vi "古田户外一体站流程质控自动启动.vi"(11 "参数":T1={"是否启用仪器"=FALSE, "CODMn"={"启动测量模式"={"测量模式"=enum."水样测量"}, "确定按钮"=TRUE}, "启动模块"={"氨氮"=FALSE, "总磷"=FALSE, "总氮"=FALSE, "COD"=FALSE}, "常规启动"=FALSE, "直接启动"=FALSE}) -> ()   [LabVIEW 2016, in "质控单元.lvlib"]
uses:
  PLC/PLC.lvlib
panel:
  out "枚举 2":enum16{"初始化", "采配水启动", "等待", "配水", "排水", "结束"}(ring)
  out "枚举":enum16{"初始化", "采配水启动", "等待", "配水", "排水", "结束"}(ring)
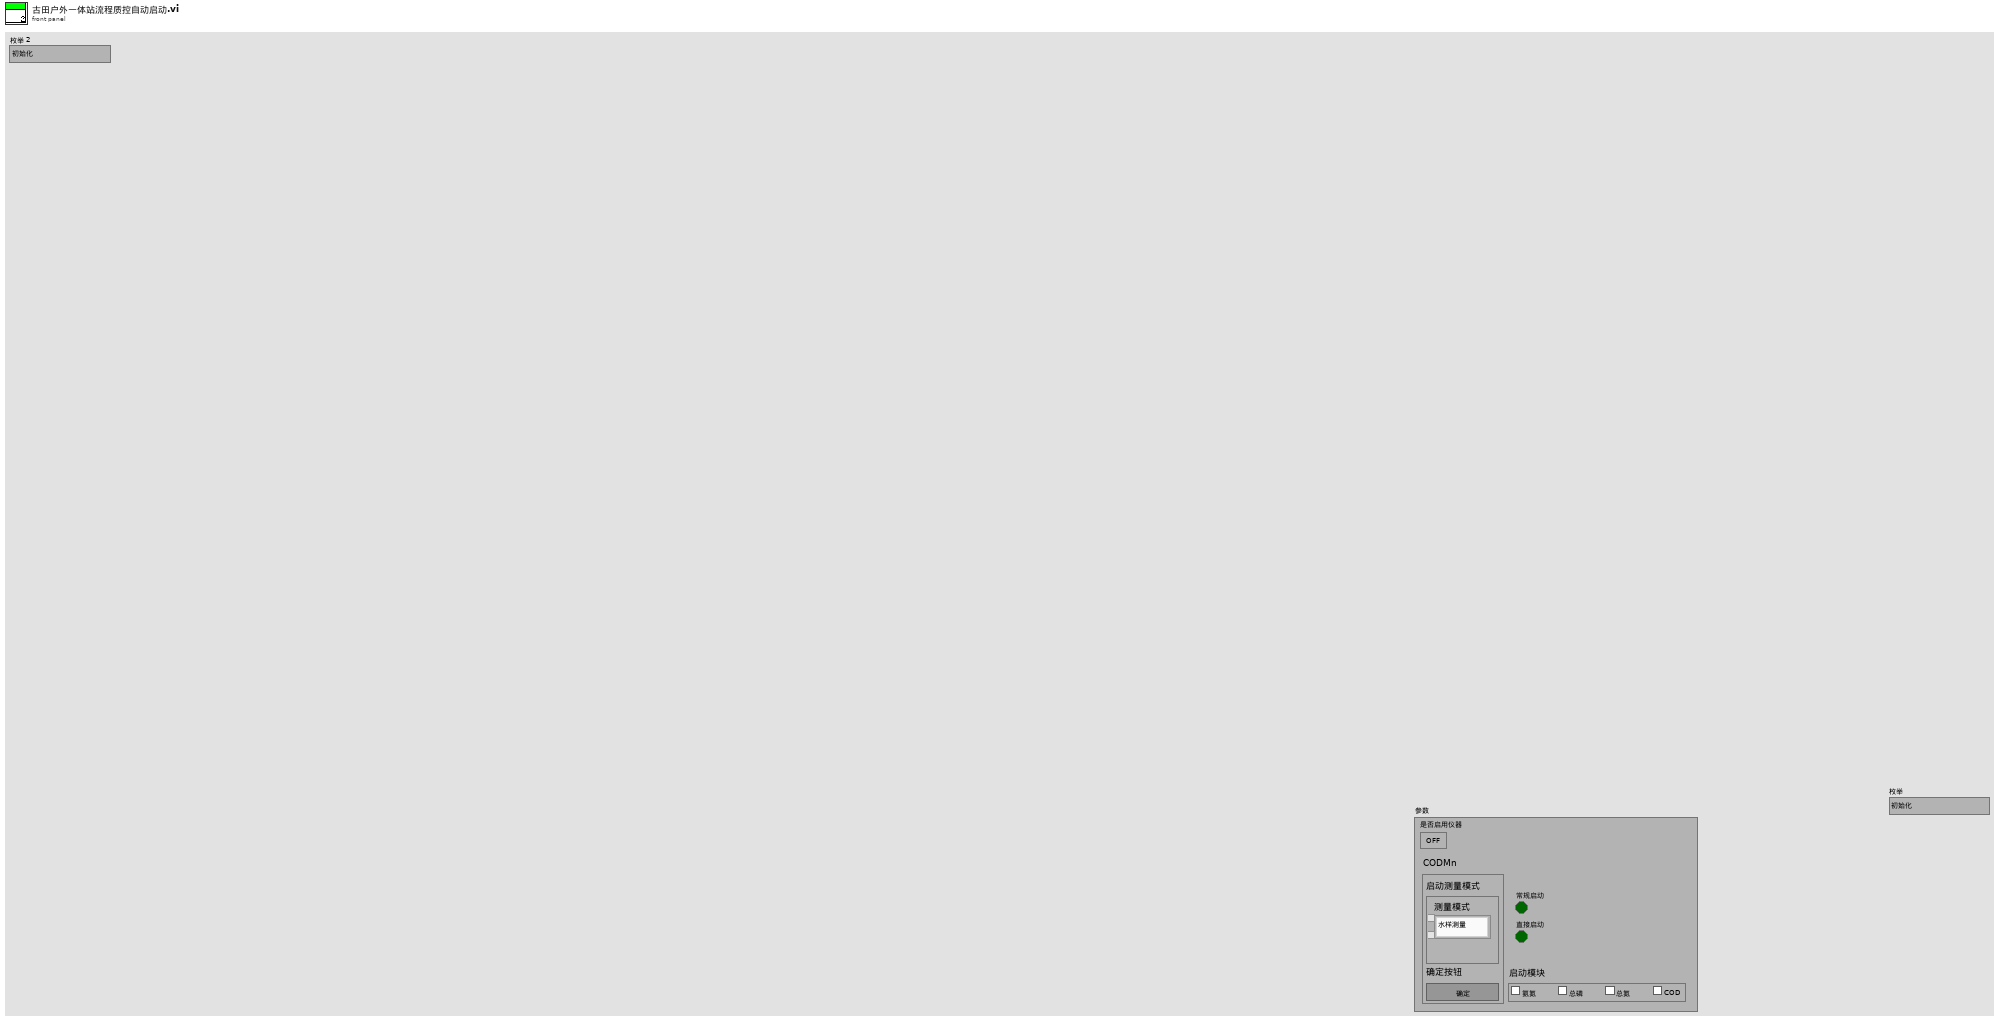
[diagram p1: front panel]
types:
  T1 = cluster{"是否启用仪器":bool, "CODMn":cluster{"启动测量模式":cluster{"测量模式":enum16{"水样测量", "标样核查", "加标回收", "平行样", "校零", "校标"}}, "确定按钮":bool}, "启动模块":cluster{"氨氮":bool, "总磷":bool, "总氮":bool, "COD":bool}, "常规启动":bool, "直接启动":bool}
  T2 = cluster{"命令":string, cluster{"starting address":u16, "holding register value":u16}}
  T3 = cluster{"R0":i16, "R1":i16, "R2":i16, "R3":i16, "R4":i16, "R5":i16, "R6":i16, "R7":i16, "R8":i16, "R9":i16, "R10":i16, "R11":i16, "R12":i16, "R13":i16, "R14":i16, "R15":i16, "R16":i16, "R17":i16, "R18":i16, "R19":i16, "R20":i16, "R21":i16}
  T4 = enum32{"Bad", "Idle", "Run top level", "Running"}
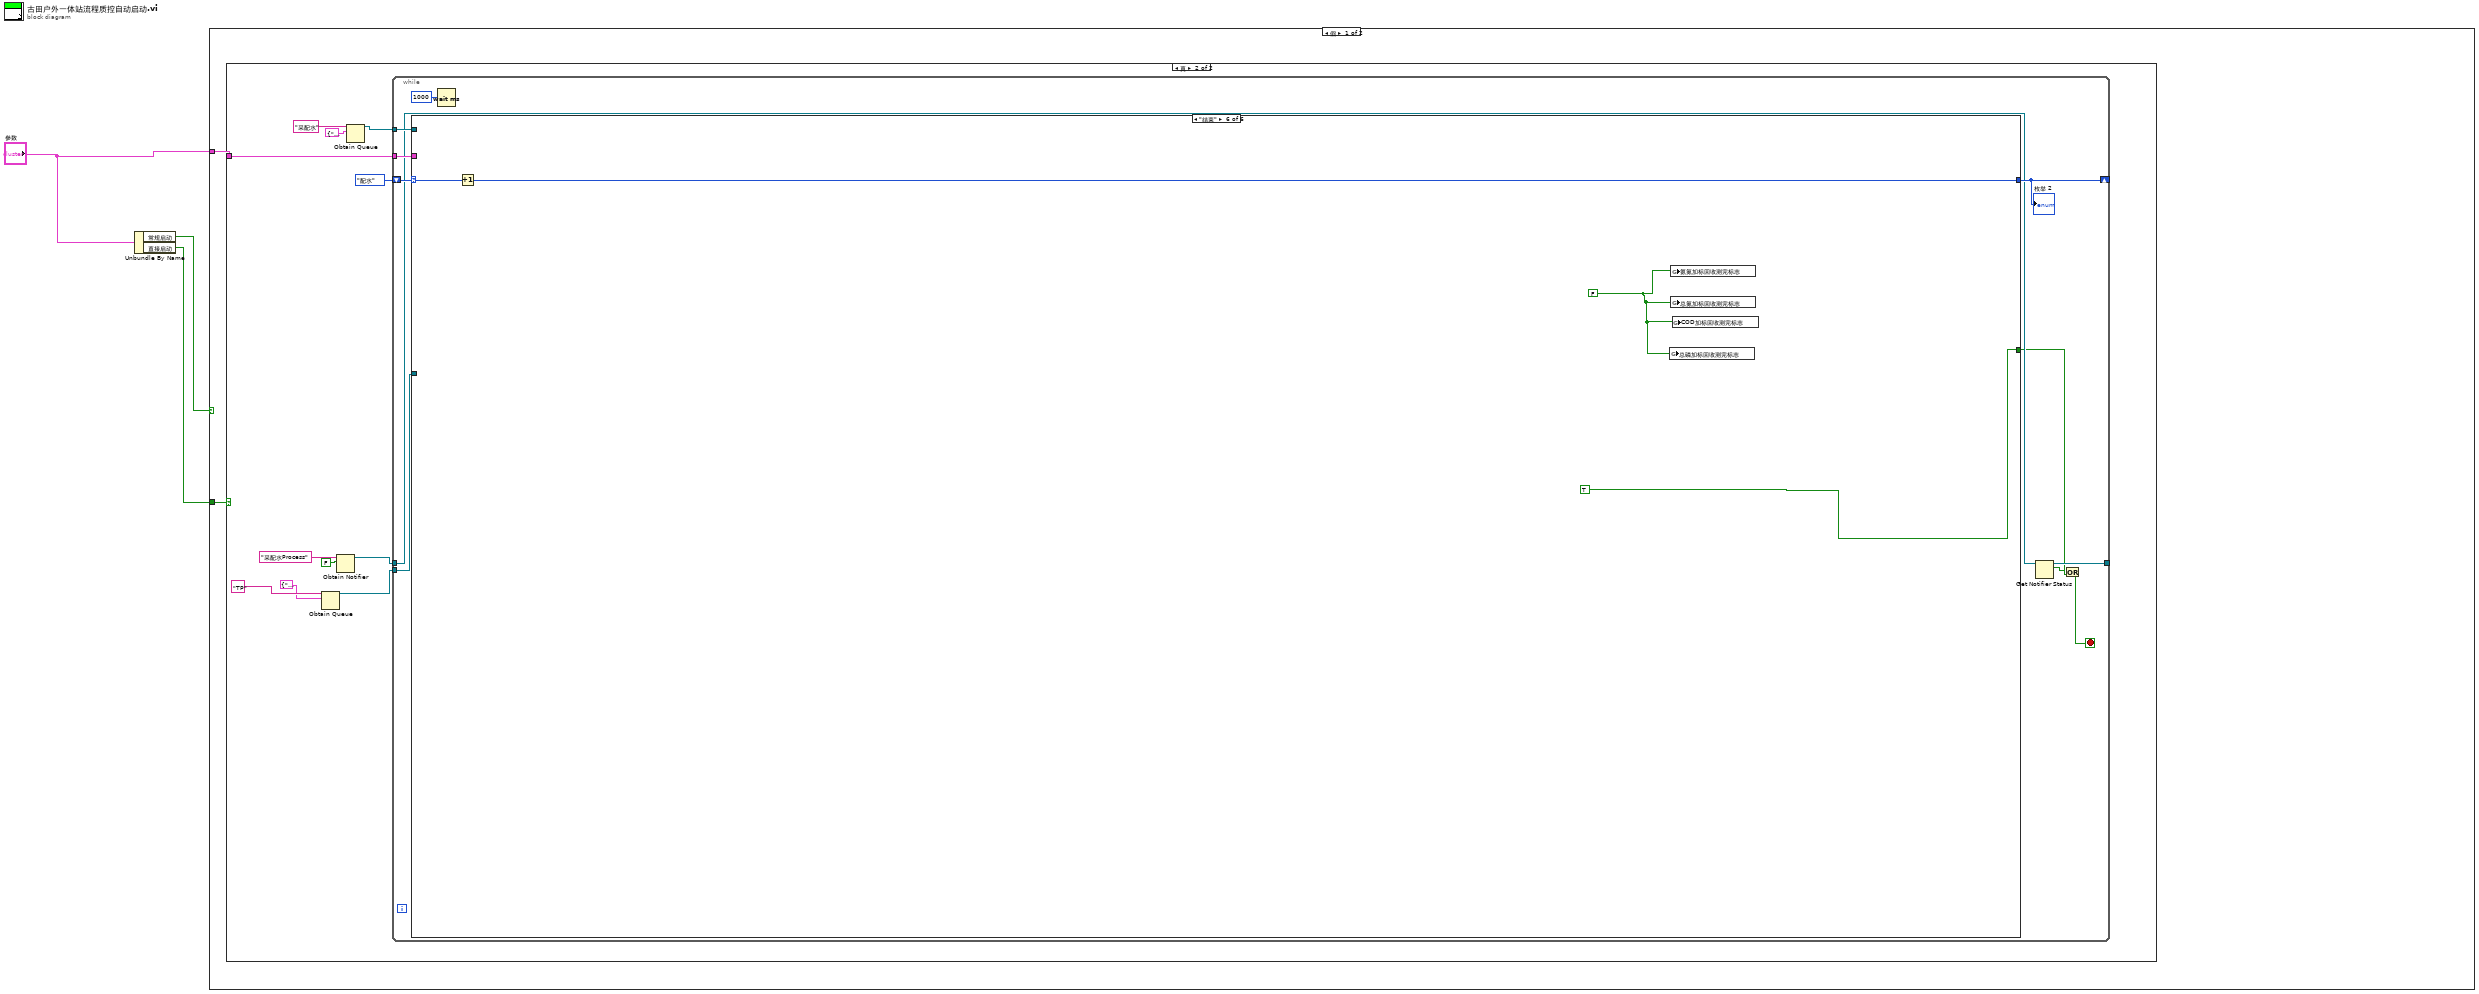
[diagram p0: block diagram]
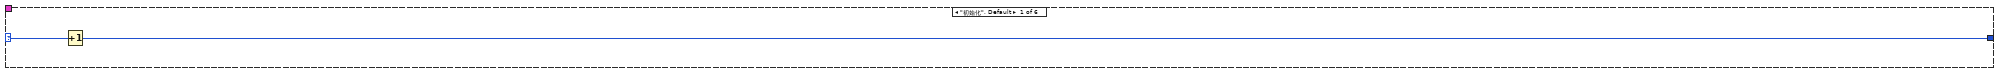
[diagram p3: hidden frame]
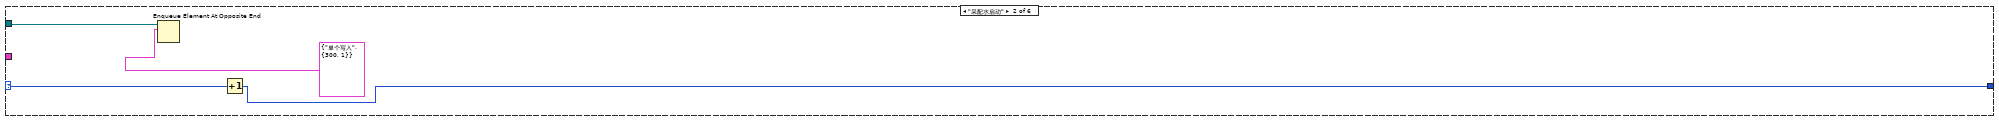
[diagram p4: hidden frame]
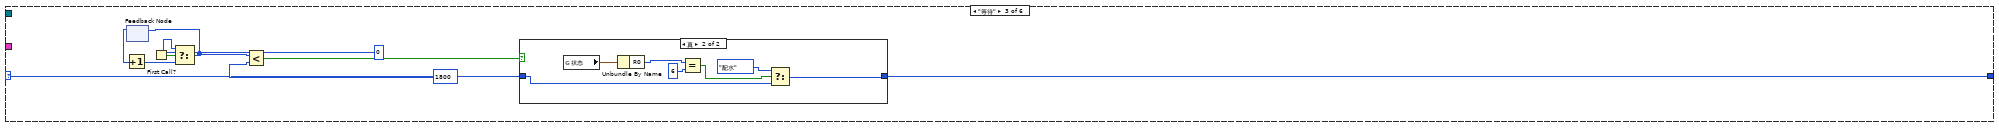
[diagram p5: hidden frame]
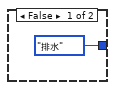
[diagram p6: hidden frame]
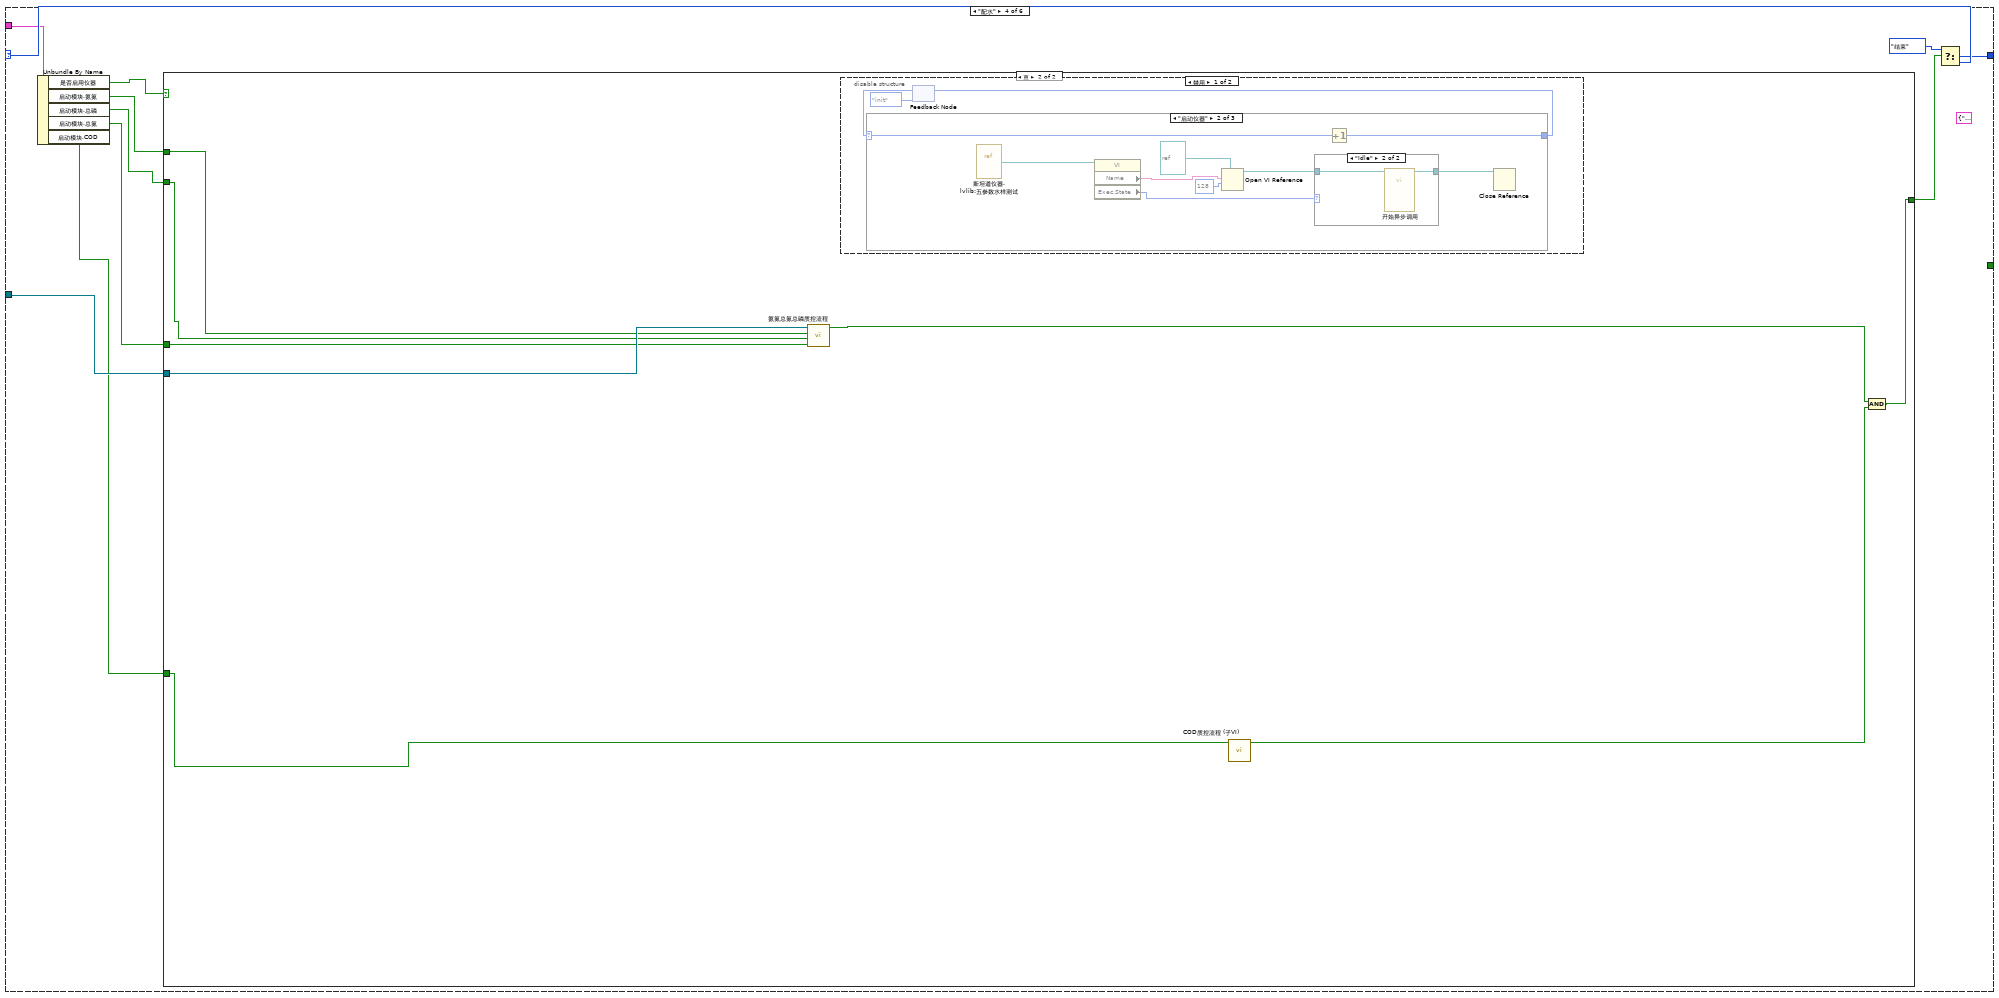
[diagram p7: hidden frame]
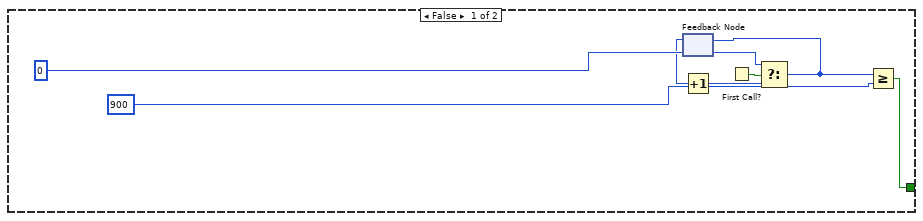
[diagram p8: hidden frame]
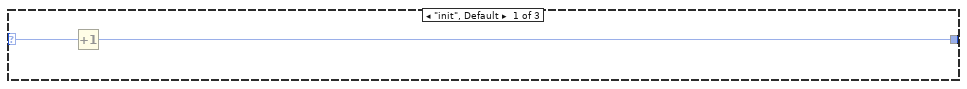
[diagram p9: hidden frame]
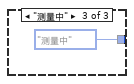
[diagram p11: hidden frame]
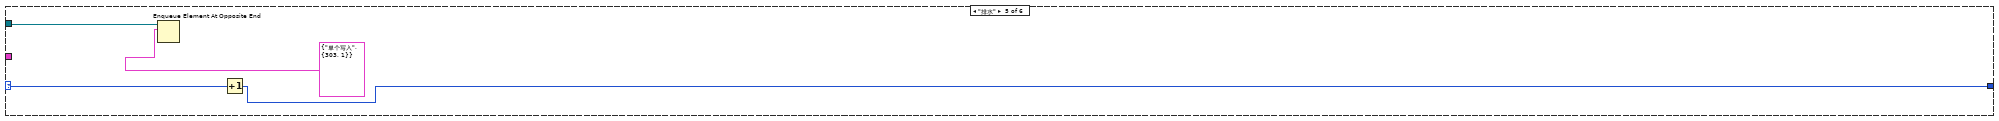
[diagram p13: hidden frame]
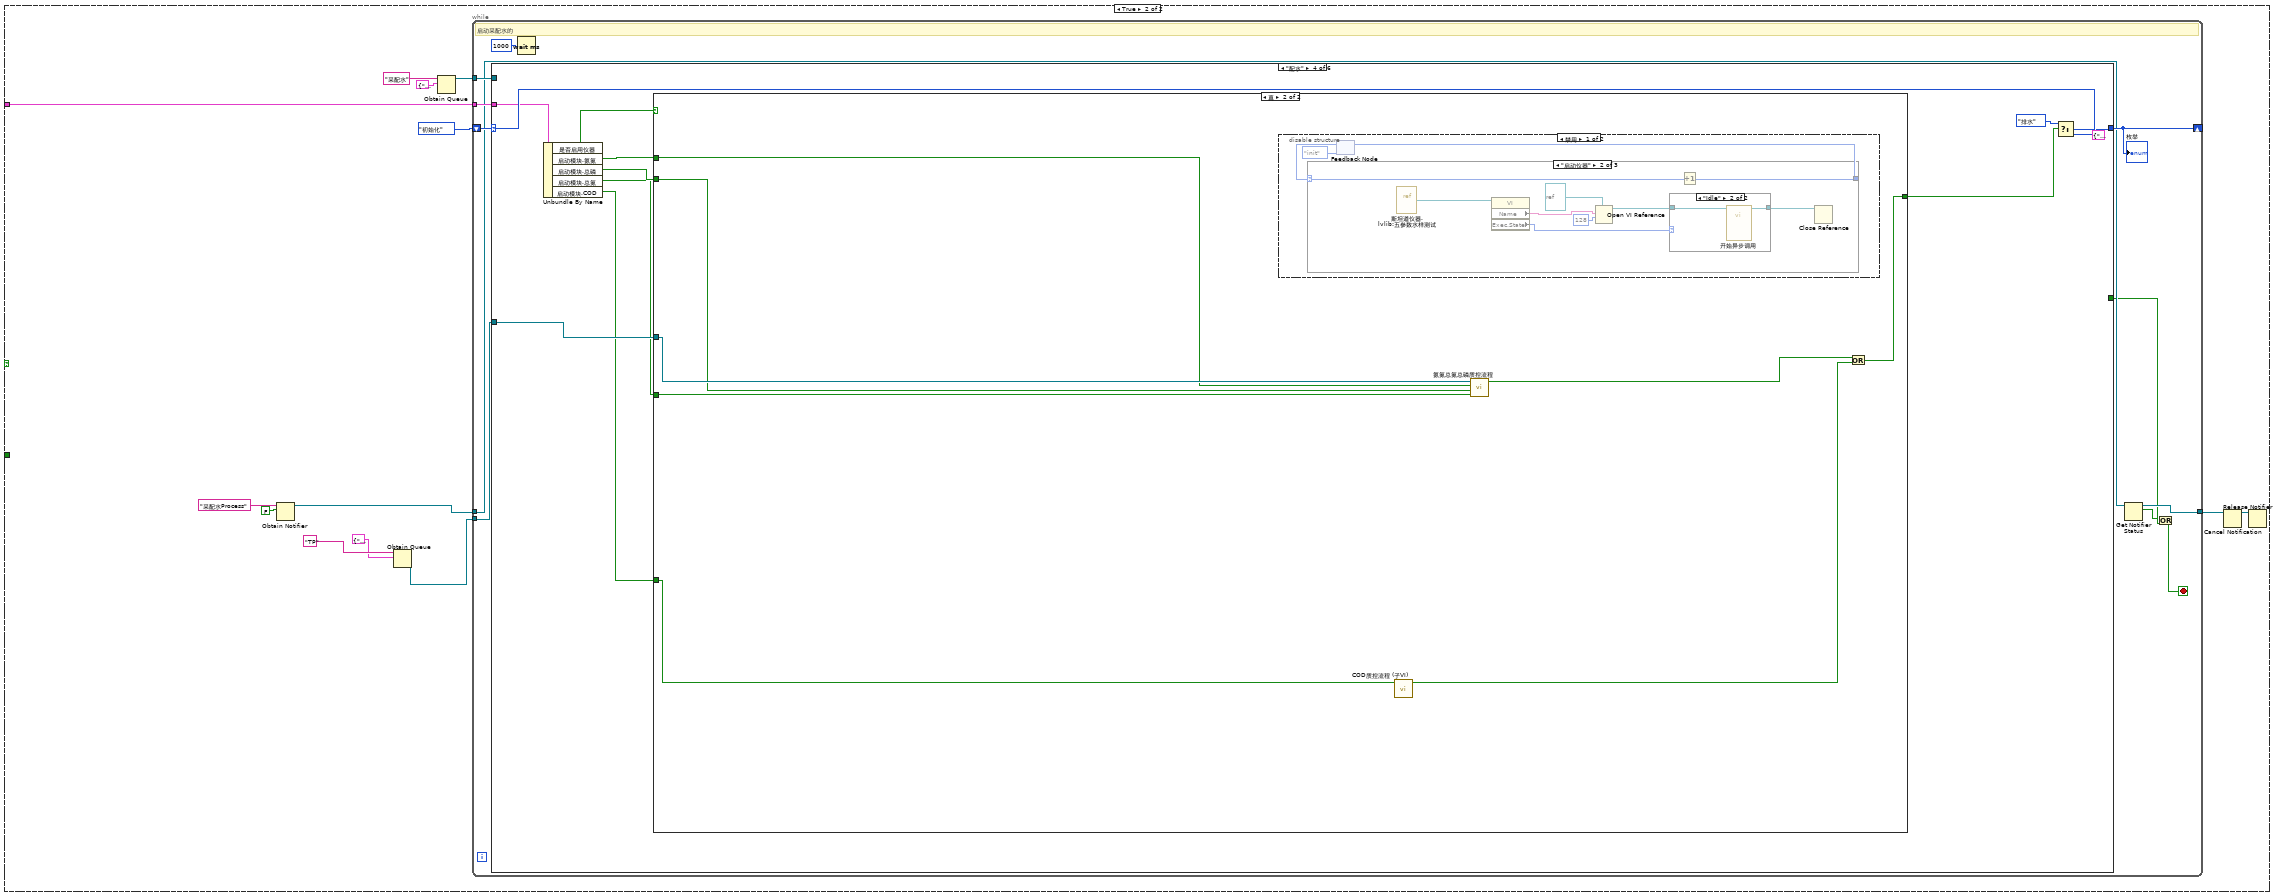
[diagram p14: hidden frame]
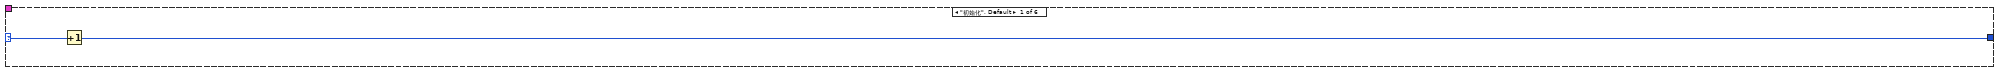
[diagram p15: hidden frame]
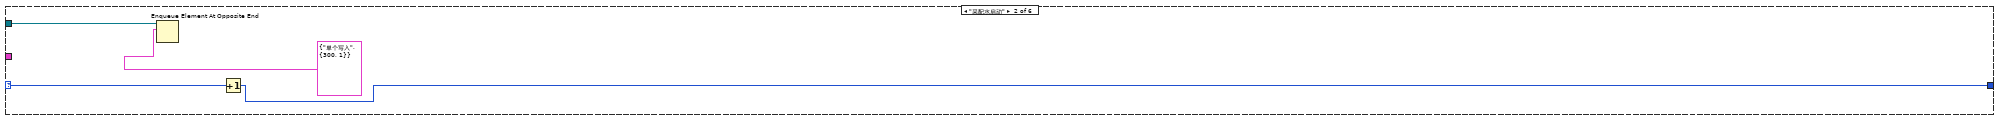
[diagram p16: hidden frame]
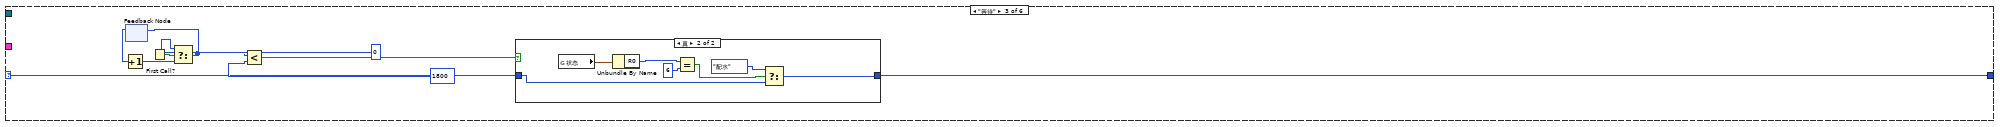
[diagram p17: hidden frame]
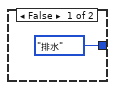
[diagram p18: hidden frame]
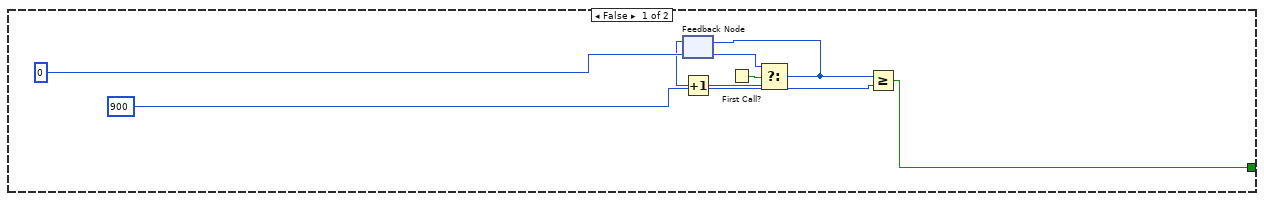
[diagram p19: hidden frame]
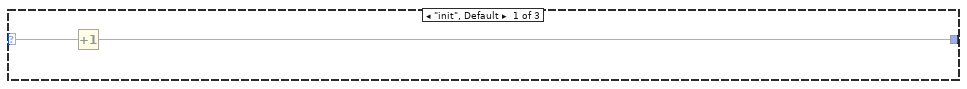
[diagram p20: hidden frame]
diagram:
  n1 = Unbundle By Name("参数") -> ("常规启动"=w2:bool, "直接启动"=w1:bool)
  n2 = case shown="假" w2 {
    tunnel: "参数" -> [w4 w103]
    tunnel: w1 -> [w5 _]
    frame False {
      n3 = case shown="真" w5 {
        tunnel: w4 -> [_ w15]
        frame False {
        }
        frame True {
          n4 = Obtain Queue(name (unnamed)="TP" ("名称（未命名）"), element data type=cluster{"命令":string, "data":variant} {"命令"="", "data"=variant}) -> (queue out=w6:refnum<queue>)  [unwired: 3 in, 2 out]
          n5 = Obtain Notifier(name (unnamed)="采配水Process" ("名称（未命名）"), notification data type=FALSE) -> (notifier out=w9:refnum<notifier>)  [unwired: 2 in, 2 out]
          n6 = Obtain Queue(name (unnamed)="采配水" ("名称（未命名）"), element data type=cluster{"命令":string, "数据":variant} {"命令"="", "数据"=variant}) -> (queue out=w12:refnum<queue>)  [unwired: 3 in, 2 out]
          n7 = while {
            tunnel: w12 -> [w27]
            shift-right: [w25] -> _
            shift-left: enum16{"初始化", "采配水启动", "等待", "配水", "排水", "结束"}."配水" ("枚举") -> [w26]
            tunnel: w6 -> [w23]
            tunnel: w15 -> [w22]
            tunnel: w9 -> [w21]
            tunnel: [w20] -> _
            stop <- w19 stop-if-true
            n8 = case shown="\"结束\"" w26 {
              selector: w26 -> [w29 w31 w40 w60 w96 w102]
              tunnel: w27 -> [_ w32 _ _ w97 _]
              tunnel: [w28 w30 w39 w59 w95 w101] -> w25
              tunnel: [_ _ _ _ _ TRUE] -> w18
              tunnel: w23 -> [_ _ _ w58 _ _]
              tunnel: w22 -> [_ _ _ w55 _ _]
              frame "初始化", Default {
                n9 = Increment(x=w29) -> (x+1=w28:enum16{"初始化", "采配水启动", "等待", "配水", "排水", "结束"})
              }
              frame "采配水启动" {
                n10 = Enqueue Element At Opposite End(queue=w32, element=T2 {"命令"="单个写入", {"starting address"=300, "holding register value"=1}} ("元素")) -> ()  [unwired: 2 in, 3 out]
                n11 = Increment(x=w31) -> (x+1=w30:enum16{"初始化", "采配水启动", "等待", "配水", "排水", "结束"})
              }
              frame "等待" {
                n12 = feedback #1() -> (w36:i32)  [unwired: 1 in]
                n13 = Increment(x=w36) -> (x+1=w35:i32)
                n14 = First Call?() -> (First Call?: T/F=w37:bool)
                n15 = Select(t=0, s=w37, f=w35) -> (s? t:f=w34:i32)
                n16 = feedback-in #1(w34) -> ()
                n17 = Less?(x=w34, y=1800) -> (x < y?=w41:bool)
                n18 = case shown="真" w41 {
                  tunnel: w40 -> [_ w45]
                  tunnel: [enum16{"初始化", "采配水启动", "等待", "配水", "排水", "结束"}."排水" ("枚举") w44] -> w39
                  frame False {
                  }
                  frame True {
                    n19 = global read "采配水全局变量.vi" "状态"() -> (w50:T3)
                    n20 = Unbundle By Name(w50) -> ("R0"=w49:i16)
                    n21 = Equal?(x=w49, y=i16 6) -> (x = y?=w47:bool)
                    n22 = Select(t=enum16{"初始化", "采配水启动", "等待", "配水", "排水", "结束"}."配水" ("枚举"), s=w47, f=w45) -> (s? t:f=w44:enum16{"初始化", "采配水启动", "等待", "配水", "排水", "结束"})
                  }
                }
              }
              frame "配水" {
                (unwired) cluster{"命令":string, "data":variant} {"命令"="启动", "data"=variant(cluster{"站号":u16, "控制命令输出":u16[]} {"站号"=1, "控制命令输出"=[256, 0]})} ("元素")
                n23 = Unbundle By Name(w55) -> ("是否启用仪器"=w57:bool, "启动模块.氨氮"=w53:bool, "启动模块.总磷"=w54:bool, "启动模块.总氮"=w51:bool, "启动模块.COD"=w52:bool)
                n24 = case shown="真" w57 {
                  tunnel: w58 -> [_ w75]
                  tunnel: [w62 w76] -> w56
                  tunnel: w54 -> [_ w73]
                  tunnel: w53 -> [_ w74]
                  tunnel: w52 -> [_ w72]
                  tunnel: w51 -> [_ w69]
                  frame False {
                    n25 = feedback #2() -> (w66:i32)  [unwired: 1 in]
                    n26 = Increment(x=w66) -> (x+1=w65:i32)
                    n27 = First Call?() -> (First Call?: T/F=w67:bool)
                    n28 = Select(t=0, s=w67, f=w65) -> (s? t:f=w63:i32)
                    n29 = feedback-in #2(w63) -> ()
                    n30 = Greater Or Equal?(x=w63, y=900) -> (x >= y?=w62:bool)
                  }
                  frame True {
                    n31 = call "氨氮总氮总磷质控流程.vi"("总氮"=w69, "总磷"=w73, "氨氮"=w74, "队列输入"=w75) -> ("布尔"=w70:bool)  [unwired: 7 in]
                    n32 = disable-structure shown="禁用" {
                      frame Disabled {
                        n33 = feedback #3(enum16{"init", "启动仪器", "测量中"}."init") -> (w78:enum16{"init", "启动仪器", "测量中"})
                        n34 = case shown="\"启动仪器\"" w78 {
                          selector: w78 -> [w81 w90 _]
                          tunnel: [w80 w89 enum16{"init", "启动仪器", "测量中"}."测量中"] -> w79
                          frame "init", Default {
                            n35 = Increment(x=w81) -> (x+1=w80:enum16{"init", "启动仪器", "测量中"})
                          }
                          frame "启动仪器" {
                            n36 = vi-ref "斯坦道仪器.lvlib:五参数水样测试.vi"() -> (w82:refnum<vi>)
                            n37 = property class="VI"(reference=w82) -> ("Name"=w86:string, "Exec.State"=w84:T4)  [unwired: 1 in, 2 out]
                            n38 = Open VI Reference(type specifier VI Refnum (for type only)=refnum<vi> refnum ("类型说明符VI引用句柄（仅用于类型）"), vi path=w86, options=128 ("选项")) -> (vi reference=w85:refnum<vi>)  [unwired: 3 in, 1 out]
                            n39 = case shown="\"Idle\"" w84 {
                              tunnel: w85 -> [w91 w93]
                              tunnel: [w91 w92] -> w83
                              frame "Bad", Default {
                              }
                              frame "Idle" {
                                n40 = call-by-ref "开始异步调用"(reference=w93) -> (reference out=w92:refnum<vi>)  [unwired: 13 in, 1 out]
                              }
                            }
                            n41 = Increment(x=w90) -> (x+1=w89:enum16{"init", "启动仪器", "测量中"})
                            n42 = Close Reference(reference=w83) -> ()  [unwired: 1 in, 1 out]
                          }
                          frame "测量中" {
                          }
                        }
                        n43 = feedback-in #3(w79) -> ()
                      }
                      frame Enabled {
                      }
                    }
                    n44 = call "COD质控流程 (子VI).vi"("COD"=w72) -> ("布尔"=w71:bool)  [unwired: 10 in]
                    n45 = And(x=w70, y=w71) -> (x .and. y?=w76:bool)
                  }
                }
                n46 = Select(t=enum16{"初始化", "采配水启动", "等待", "配水", "排水", "结束"}."结束" ("枚举"), s=w56, f=w60) -> (s? t:f=w59:enum16{"初始化", "采配水启动", "等待", "配水", "排水", "结束"})
              }
              frame "排水" {
                n47 = Enqueue Element At Opposite End(queue=w97, element=T2 {"命令"="单个写入", {"starting address"=303, "holding register value"=1}} ("元素")) -> ()  [unwired: 2 in, 3 out]
                n48 = Increment(x=w96) -> (x+1=w95:enum16{"初始化", "采配水启动", "等待", "配水", "排水", "结束"})
              }
              frame "结束" {
                w99 = FALSE ("氨氮加标回收测完标志")
                n49 = Increment(x=w102) -> (x+1=w101:enum16{"初始化", "采配水启动", "等待", "配水", "排水", "结束"})
                n50 = global write "质控测完标志全局 1.vi" "总磷加标回收测完标志"(w99) -> ()
                n51 = global write "质控测完标志全局 1.vi" "氨氮加标回收测完标志"(w99) -> ()
                n52 = global write "质控测完标志全局 1.vi" "总氮加标回收测完标志"(w99) -> ()
                n53 = global write "质控测完标志全局 1.vi" "COD加标回收测完标志"(w99) -> ()
              }
            }
            "枚举 2" <- w25
            n54 = Wait (ms)(milliseconds to wait=u32 1000 ("等待时间（毫秒）")) -> ()  [unwired: 1 out]
            n55 = Get Notifier Status(notifier=w21) -> (notifier out=w20:refnum<notifier>, current notification=w17:bool)  [unwired: 1 in, 3 out]
            n56 = Or(x=w17, y=w18) -> (x .or. y?=w19:bool)
          }
        }
      }
    }
    frame True {
      n57 = Obtain Notifier(name (unnamed)="采配水Process" ("名称（未命名）"), notification data type=FALSE) -> (notifier out=w106:refnum<notifier>)  [unwired: 2 in, 2 out]
      n58 = Obtain Queue(name (unnamed)="TP" ("名称（未命名）"), element data type=cluster{"命令":string, "data":variant} {"命令"="", "data"=variant}) -> (queue out=w109:refnum<queue>)  [unwired: 3 in, 2 out]
      n59 = Obtain Queue(name (unnamed)="采配水" ("名称（未命名）"), element data type=cluster{"命令":string, "数据":variant} {"命令"="", "数据"=variant}) -> (queue out=w113:refnum<queue>)  [unwired: 3 in, 2 out]
      n60 = while {
        tunnel: w113 -> [w126]
        shift-right: [w124] -> _
        shift-left: enum16{"初始化", "采配水启动", "等待", "配水", "排水", "结束"}."初始化" ("枚举") -> [w125]
        tunnel: w109 -> [w122]
        tunnel: w103 -> [w121]
        tunnel: w106 -> [w120]
        tunnel: [w119] -> w105
        stop <- w118 stop-if-true
        # "启动采配水的"
        n61 = case shown="\"配水\"" w125 {
          selector: w125 -> [w128 w130 w139 w159 w195 w200]
          tunnel: w126 -> [_ w131 _ _ w196 _]
          tunnel: [w127 w129 w138 w158 w194 w199] -> w124
          tunnel: [_ _ _ _ _ TRUE] -> w117
          tunnel: w122 -> [_ _ _ w157 _ _]
          tunnel: w121 -> [_ _ _ w154 _ _]
          frame "初始化", Default {
            n62 = Increment(x=w128) -> (x+1=w127:enum16{"初始化", "采配水启动", "等待", "配水", "排水", "结束"})
          }
          frame "采配水启动" {
            n63 = Enqueue Element At Opposite End(queue=w131, element=T2 {"命令"="单个写入", {"starting address"=300, "holding register value"=1}} ("元素")) -> ()  [unwired: 2 in, 3 out]
            n64 = Increment(x=w130) -> (x+1=w129:enum16{"初始化", "采配水启动", "等待", "配水", "排水", "结束"})
          }
          frame "等待" {
            n65 = feedback #4() -> (w135:i32)  [unwired: 1 in]
            n66 = Increment(x=w135) -> (x+1=w134:i32)
            n67 = First Call?() -> (First Call?: T/F=w136:bool)
            n68 = Select(t=0, s=w136, f=w134) -> (s? t:f=w133:i32)
            n69 = feedback-in #4(w133) -> ()
            n70 = Less?(x=w133, y=1800) -> (x < y?=w140:bool)
            n71 = case shown="真" w140 {
              tunnel: w139 -> [_ w144]
              tunnel: [enum16{"初始化", "采配水启动", "等待", "配水", "排水", "结束"}."排水" ("枚举") w143] -> w138
              frame False {
              }
              frame True {
                n72 = global read "采配水全局变量.vi" "状态"() -> (w149:T3)
                n73 = Unbundle By Name(w149) -> ("R0"=w148:i16)
                n74 = Equal?(x=w148, y=i16 6) -> (x = y?=w146:bool)
                n75 = Select(t=enum16{"初始化", "采配水启动", "等待", "配水", "排水", "结束"}."配水" ("枚举"), s=w146, f=w144) -> (s? t:f=w143:enum16{"初始化", "采配水启动", "等待", "配水", "排水", "结束"})
              }
            }
          }
          frame "配水" {
            (unwired) cluster{"命令":string, "data":variant} {"命令"="启动", "data"=variant(cluster{"站号":u16, "控制命令输出":u16[]} {"站号"=1, "控制命令输出"=[256, 0]})} ("元素")
            n76 = Unbundle By Name(w154) -> ("是否启用仪器"=w156:bool, "启动模块.氨氮"=w152:bool, "启动模块.总磷"=w153:bool, "启动模块.总氮"=w150:bool, "启动模块.COD"=w151:bool)
            n77 = case shown="真" w156 {
              tunnel: w157 -> [_ w175]
              tunnel: [w161 w172] -> w155
              tunnel: w153 -> [_ w171]
              tunnel: w152 -> [_ w170]
              tunnel: w151 -> [_ w169]
              tunnel: w150 -> [_ w168]
              frame False {
                n78 = feedback #5() -> (w165:i32)  [unwired: 1 in]
                n79 = Increment(x=w165) -> (x+1=w164:i32)
                n80 = First Call?() -> (First Call?: T/F=w166:bool)
                n81 = Select(t=0, s=w166, f=w164) -> (s? t:f=w162:i32)
                n82 = feedback-in #5(w162) -> ()
                n83 = Greater Or Equal?(x=w162, y=900) -> (x >= y?=w161:bool)
              }
              frame True {
                n84 = disable-structure shown="禁用" {
                  frame Disabled {
                    n85 = feedback #6(enum16{"init", "启动仪器", "测量中"}."init") -> (w177:enum16{"init", "启动仪器", "测量中"})
                    n86 = case shown="\"启动仪器\"" w177 {
                      selector: w177 -> [w180 w189 _]
                      tunnel: [w179 w188 enum16{"init", "启动仪器", "测量中"}."测量中"] -> w178
                      frame "init", Default {
                        n87 = Increment(x=w180) -> (x+1=w179:enum16{"init", "启动仪器", "测量中"})
                      }
                      frame "启动仪器" {
                        n88 = vi-ref "斯坦道仪器.lvlib:五参数水样测试.vi"() -> (w181:refnum<vi>)
                        n89 = property class="VI"(reference=w181) -> ("Name"=w185:string, "Exec.State"=w183:T4)  [unwired: 1 in, 2 out]
                        n90 = Open VI Reference(type specifier VI Refnum (for type only)=refnum<vi> refnum ("类型说明符VI引用句柄（仅用于类型）"), vi path=w185, options=128 ("选项")) -> (vi reference=w184:refnum<vi>)  [unwired: 3 in, 1 out]
                        n91 = case shown="\"Idle\"" w183 {
                          tunnel: w184 -> [w190 w192]
                          tunnel: [w190 w191] -> w182
                          frame "Bad", Default {
                          }
                          frame "Idle" {
                            n92 = call-by-ref "开始异步调用"(reference=w192) -> (reference out=w191:refnum<vi>)  [unwired: 13 in, 1 out]
                          }
                        }
                        n93 = Increment(x=w189) -> (x+1=w188:enum16{"init", "启动仪器", "测量中"})
                        n94 = Close Reference(reference=w182) -> ()  [unwired: 1 in, 1 out]
                      }
                      frame "测量中" {
                      }
                    }
                    n95 = feedback-in #6(w178) -> ()
                  }
                  frame Enabled {
                  }
                }
                n96 = call "COD质控流程 (子VI).vi"("COD"=w169) -> ("布尔"=w173:bool)  [unwired: 10 in]
                n97 = call "氨氮总氮总磷质控流程.vi"("总氮"=w168, "总磷"=w171, "氨氮"=w170, "队列输入"=w175) -> ("布尔"=w174:bool)  [unwired: 7 in]
                n98 = Or(x=w174, y=w173) -> (x .or. y?=w172:bool)
              }
            }
            n99 = Select(t=enum16{"初始化", "采配水启动", "等待", "配水", "排水", "结束"}."排水" ("枚举"), s=w155, f=w159) -> (s? t:f=w158:enum16{"初始化", "采配水启动", "等待", "配水", "排水", "结束"})
          }
          frame "排水" {
            n100 = Enqueue Element At Opposite End(queue=w196, element=T2 {"命令"="单个写入", {"starting address"=303, "holding register value"=1}} ("元素")) -> ()  [unwired: 2 in, 3 out]
            n101 = Increment(x=w195) -> (x+1=w194:enum16{"初始化", "采配水启动", "等待", "配水", "排水", "结束"})
          }
          frame "结束" {
            n102 = Increment(x=w200) -> (x+1=w199:enum16{"初始化", "采配水启动", "等待", "配水", "排水", "结束"})
          }
        }
        "枚举" <- w124
        n103 = Wait (ms)(milliseconds to wait=u32 1000 ("等待时间（毫秒）")) -> ()  [unwired: 1 out]
        n104 = Get Notifier Status(notifier=w120) -> (notifier out=w119:refnum<notifier>, current notification=w116:bool)  [unwired: 1 in, 3 out]
        n105 = Or(x=w116, y=w117) -> (x .or. y?=w118:bool)
      }
      n106 = Cancel Notification(0:w105) -> (8:w104:refnum<notifier>)  [unwired: 1 in, 2 out]
      n107 = Release Notifier(notifier=w104) -> ()  [unwired: 2 in, 3 out]
    }
  }
